vi "testmyrio.vi"() -> ()   [LabVIEW 2014]
uses:
  <vilib>/Platform/TimedLoop/XDataNode/timing_clust.ctl
  <vilib>/Platform/TimedLoop/XDataNode/nitl_modes.ctl
  <vilib>/Platform/TimedLoop/XDataNode/wakeup.ctl
  <vilib>/myRIO/Common/Instrument Driver Framework/myRIO v1.0/PWM/vis/myRIO v1.1 Open PWM.vi
  <vilib>/myRIO/Common/Instrument Driver Framework/Utilities/vis/Validate Channels.vi
  <vilib>/myRIO/Common/Instrument Driver Framework/myRIO v1.0/PWM/vis/myRIO v1.0 Reserve PWM.vi
  <vilib>/myRIO/Common/Instrument Driver Framework/myRIO v1.0/PWM/vis/myRIO v1.0 Build MUX Configuration PWM.vi
  <vilib>/myRIO/Common/Instrument Driver Framework/myRIO v1.0/Resource Manager/vis/myRIO v1.0 Reserve Channel List.vi
  <vilib>/myRIO/Common/Instrument Driver Framework/myRIO v1.0/Resource Manager/vis/myRIO v1.0 Create Configuration List.vi
  <vilib>/myRIO/Common/Instrument Driver Framework/myRIO v1.0/Resource Manager/vis/myRIO v1.0 Reserve Channel.vi
  <vilib>/myRIO/Common/Instrument Driver Framework/myRIO v1.0/Resource Manager/vis/myRIO v1.0 Unreserve Channel.vi
  <vilib>/myRIO/Common/Instrument Driver Framework/myRIO v1.0/Resource Manager/vis/myRIO v1.0 Build Mutex Name.vi
  <vilib>/Utility/VariantDataType/GetNumericInfo.vi
  <vilib>/Utility/error.llb/Error Cluster From Error Code.vi
  <vilib>/myRIO/Common/Instrument Driver Framework/myRIO v1.0/myRIO v1.1 Open.vi
  <vilib>/myRIO/Common/Instrument Driver Framework/Utilities/vis/IO Manager.vi
  <vilib>/myRIO/Common/Instrument Driver Framework/Utilities/vis/Configuration Manager.vi
  <vilib>/myRIO/Common/Instrument Driver Framework/myRIO v1.0/Resource Manager/vis/myRIO v1.0 Configure IO.vi
  <vilib>/myRIO/Common/Instrument Driver Framework/myRIO v1.0/myRIO v1.0 Close.vi
  <vilib>/Utility/AngleManip/Degrees to Radians (Scalar DBL).vi
  <vilib>/myRIO/Common/Instrument Driver Framework/myRIO v1.0/PWM/vis/myRIO v1.0 Write PWM.vi
  <vilib>/Platform/TimedLoop/XDataNode/XDataNode.xnode
  <vilib>/Platform/TimedLoop/XDataNode/XDNodeRunTimeDep.lvlib
  <vilib>/Utility/AngleManip/NI_AngleManipulation.lvlib
  <vilib>/myRIO/Instrument Drivers/Onboard IO/PWM/PWM.lvlib
panel:
  in  "Knob":dbl(knob)=125.18911398343852 scale=-180.0..180.0
  in  "open/close":dbl(slide)=-99.18367346938776 scale=-180.0..180.0
  out "theta3":dbl
  out "x/y 4":dbl
  out "x/y 3":dbl
  out "x/y 2":dbl
  out "x/y":dbl
  out "s? t:f":dbl[](array[numeric])
  in  "stop":bool
  in  "theta":dbl(knob) scale=-180.0..180.0
  in  "X":dbl(slide)=4.08910891089109 scale=0.0..11.0
  in  "Y":dbl(slide)=4.790575916230366 scale=0.0..11.9
  out "Invalid Position":bool
  out "appended array":dbl[](array[numeric])
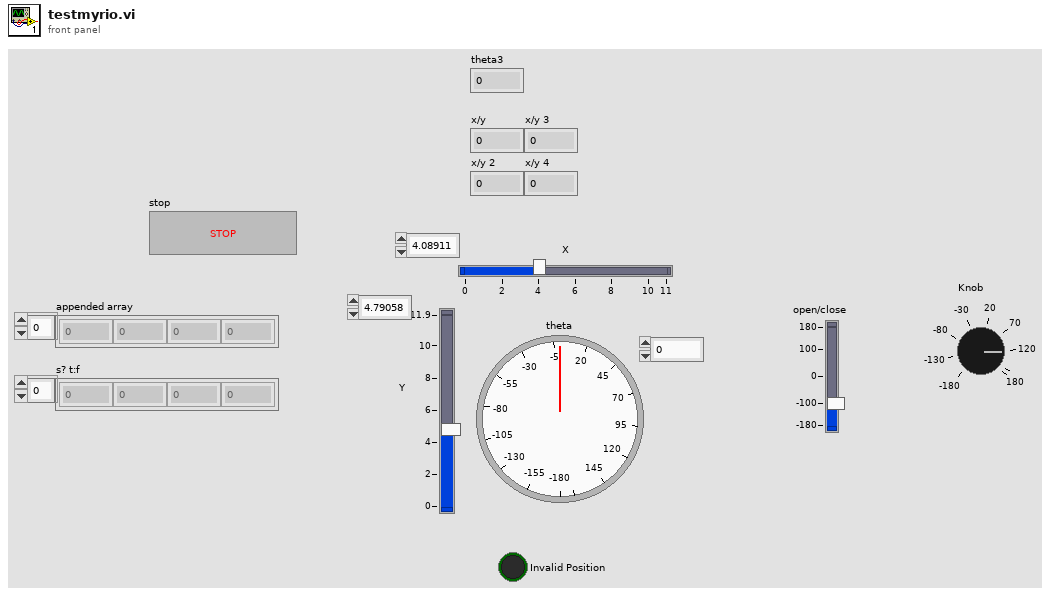
[diagram p1: front panel]
types:
  T1 = typedef "PWM.lvlib/PWM Reference.ctl" = cluster{"myRIO Reference":T2, "PWM Channels Enum":T6, "PWM Configuration":T7}
  T2 = typedef "myRIO Generic Hardware Reference.ctl" = cluster{"myRIO Model":T3, "myRIO Hardware Reference":T4}
  T3 = typedef "Hardware Version Enum.ctl" = enum16{"Unknown", "myRIO-1900", "myRIO-1950"}
  T4 = typedef "myRIO v1.0 Reference.ctl" = cluster{"Generic FPGA Reference":T5, "Allow multiple opens":bool}
  T5 = typedef "Generic FPGA Reference.ctl" = refnum<k20>
  T6 = typedef "PWM Channels Enum.ctl" = enum16{"Not Connected", "C/PWM0", "C/PWM1", "A/PWM0", "A/PWM1", "A/PWM2", "B/PWM0", "B/PWM1", "B/PWM2"}
  T7 = typedef "PWM.lvlib/PWM Configuration.ctl" = cluster{"Frequency":dbl, "Duty Cycle":dbl}
  T8 = typedef "XDNodeRunTimeDep.lvlib/timing_clust.ctl" = cluster{"Expected End [f-1]":u64, "Actual End [f-1]":u64, "Finished Late? [f-1]":bool, "Expected End [i-1]":u64, "Actual End [i-1]":u64, "Finished Late? [i-1]":bool, "Expected Start [i]":u64, "Actual Start [i]":u64, "Expected Start [f]":u64, "Actual Start [f]":u64, "Source Name":string, "Structure Name":string, "Period":i64, "Deadline":i64, "Offset":i64, "Start":i64, "Priority":i32, "Timeout":i32, "Mode":T9, "Wakeup Reason":T10, "Error":errorcluster, "Source Type":string, "Secondary Source Type":string, "Global End Time":u64, "Global Start Time":u64, "Frame Duration":u64, "Iteration Duration":u64, "Assigned CPU":i32, "I/O Scan Engine Mode":u32}
  T9 = typedef "XDNodeRunTimeDep.lvlib/nitl_modes.ctl" = enum32{"No Change", "Process missed periods, maintain original phase", "Discard missed periods, maintain original phase", "Process missed periods, ignore original phase", "Discard missed periods, ignore original phase"}
  T10 = typedef "XDNodeRunTimeDep.lvlib/wakeup.ctl" = enum32{"Normal", "Aborted", "Asynchronous wakeup", "Timing source error", "Timed loop error", "Timeout"}
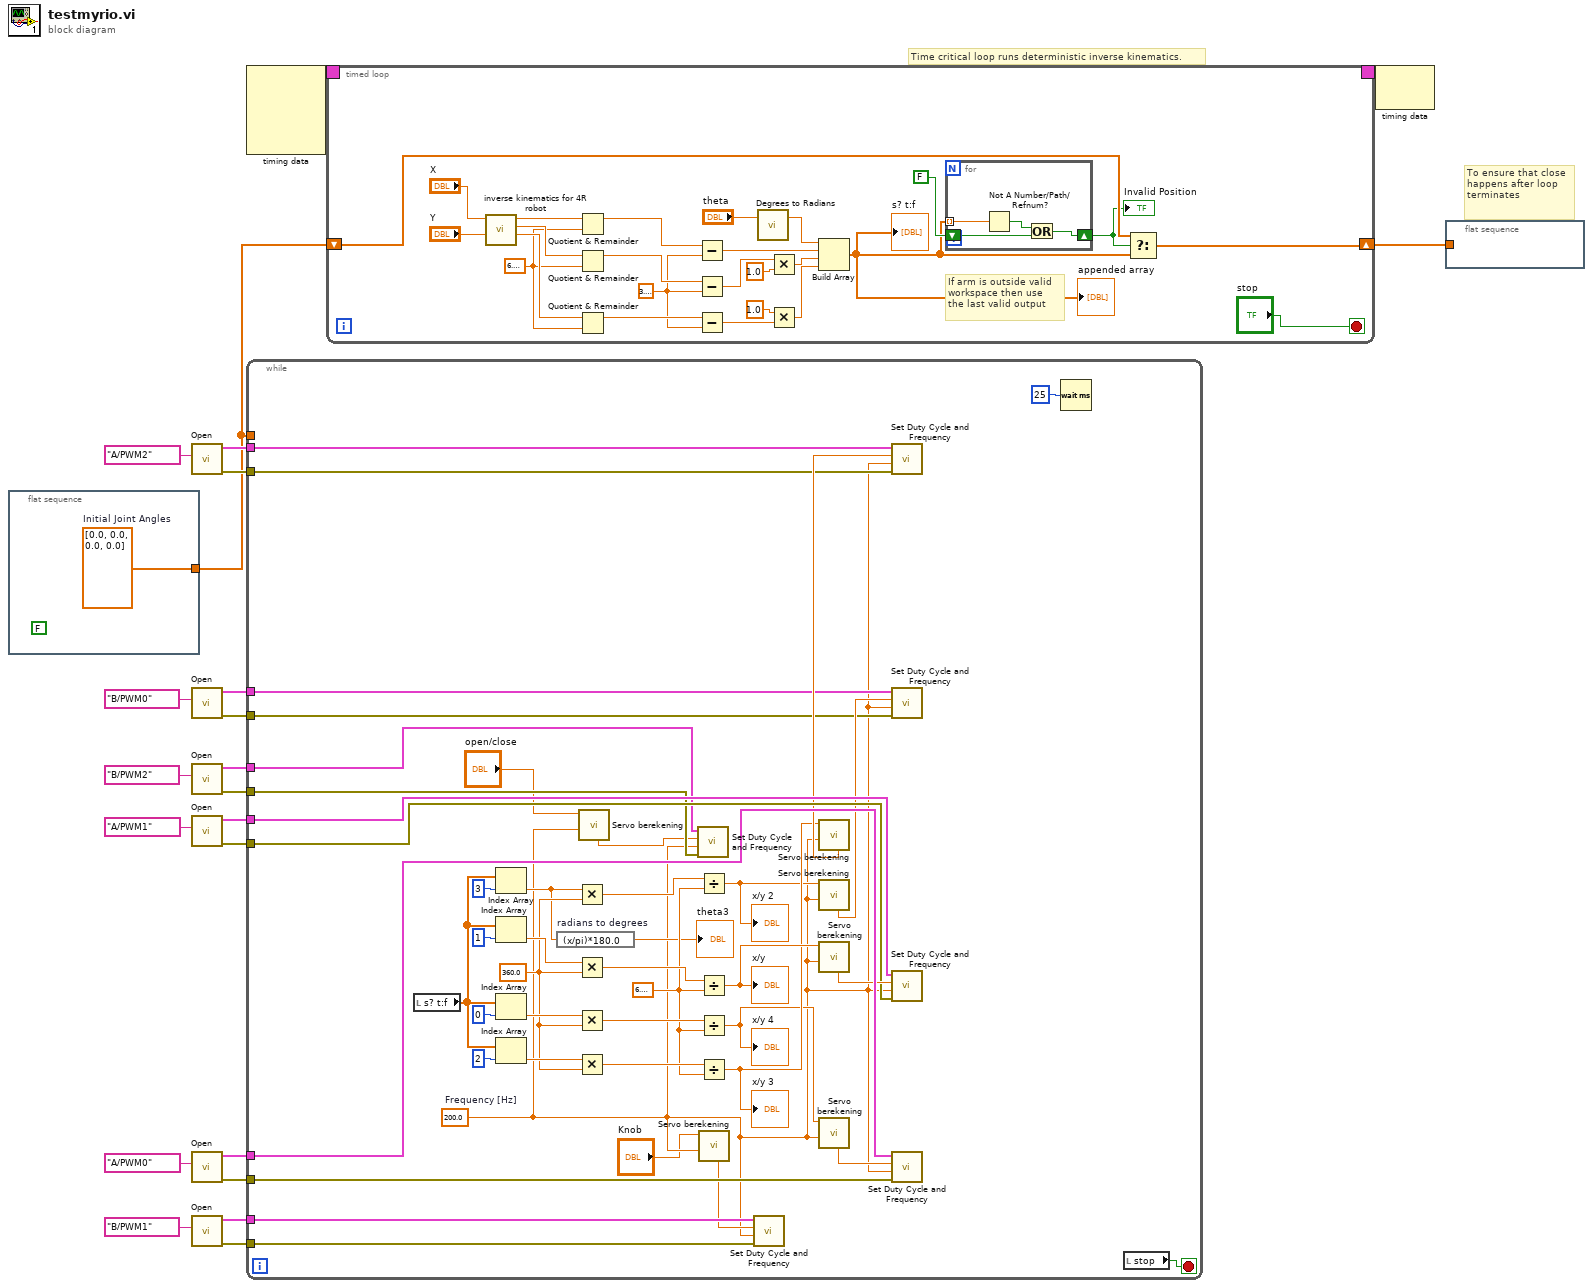
[diagram p0: block diagram]
diagram:
  # "To ensure that close happens after loop terminates"
  # "Time critical loop runs deterministic inverse kinematics."
  n1 = flat-sequence {
    tunnel: [w23] -> w7
    frame #0 {
      (unwired) FALSE ("stop")
      w23 = dbl[] [0.0, 0.0, 0.0, 0.0]  # Initial Joint Angles
    }
  }
  n2 = call <vilib>:"Open.vi"("Channel Name"=tag "A/PWM2") -> ("error out"=w11:errorcluster, "PWM Ref Out"=w12:T1)  [unwired: 9 in]
  n3 = call <vilib>:"Open.vi"("Channel Name"=tag "B/PWM0") -> ("error out"=w8:errorcluster, "PWM Ref Out"=w9:T1)  [unwired: 9 in]
  n4 = call <vilib>:"Open.vi"("Channel Name"=tag "B/PWM2") -> ("error out"=w4:errorcluster, "PWM Ref Out"=w5:T1)  [unwired: 9 in]
  n5 = call <vilib>:"Open.vi"("Channel Name"=tag "A/PWM1") -> ("error out"=w14:errorcluster, "PWM Ref Out"=w15:T1)  [unwired: 9 in]
  n6 = call <vilib>:"Open.vi"("Channel Name"=tag "A/PWM0") -> ("error out"=w18:errorcluster, "PWM Ref Out"=w19:T1)  [unwired: 9 in]
  n7 = call <vilib>:"Open.vi"("Channel Name"=tag "B/PWM1") -> ("error out"=w1:errorcluster, "PWM Ref Out"=w2:T1)  [unwired: 9 in]
  n8 = node-c288() -> (w22:T8)  [unwired: 4 in]
  n9 = while {
    tunnel: w19 -> [w62]
    tunnel: w18 -> [w61]
    tunnel: w15 -> [w59]
    tunnel: w14 -> [w58]
    tunnel: w12 -> [w55]
    tunnel: w11 -> [w54]
    tunnel: w9 -> [w51]
    tunnel: w8 -> [w50]
    tunnel: w7 -> [_]
    tunnel: w5 -> [w32]
    tunnel: w4 -> [w31]
    tunnel: w2 -> [w28]
    tunnel: w1 -> [w27]
    stop <- w33 stop-if-true
    w37 = 6.283185307179586
    w38 = 360.0 ("y")
    w25 = 200.0  # Frequency [Hz]
    n10 = local read "s? t:f"() -> (w49:dbl[])
    n11 = Index Array(array=w49, index=3) -> (element=w35:dbl)
    n12 = Index Array(array=w49, index=1) -> (element=w44:dbl)
    n13 = Index Array(array=w49, index=0) -> (element=w40:dbl)
    n14 = Index Array(array=w49, index=2) -> (element=w42:dbl)
    n15 = expression code="(x/pi)*180.0" "radians to degrees"(w35) -> (→"theta3":dbl)
    n16 = Multiply(x=w35, y=w38) -> (x*y=w46:dbl)
    n17 = Multiply(x=w44, y=w38) -> (x*y=w48:dbl)
    n18 = Multiply(x=w40, y=w38) -> (x*y=w45:dbl)
    n19 = Multiply(x=w42, y=w38) -> (x*y=w47:dbl)
    n20 = call "Servo berekening.vi"("freq [Hz]"=w25, "position [%FS] in"="open/close") -> ("Duty Cycle"=w30:dbl)  [unwired: 6 in, 3 out]
    n21 = call <vilib>:"Set Duty Cycle and Frequency.vi"("error in (no error)"=w31, "Frequency [Hz]"=w25, "Duty Cycle"=w30, "PWM Ref In"=w32) -> ()  [unwired: 5 in, 2 out]
    n22 = Divide(x=w46, y=w37) -> (x/y=w39:dbl)
    "x/y 2" <- w39
    n23 = Divide(x=w48, y=w37) -> (x/y=w43:dbl)
    "x/y" <- w43
    n24 = Divide(x=w45, y=w37) -> (x/y=w36:dbl)
    "x/y 4" <- w36
    n25 = Divide(x=w47, y=w37) -> (x/y=w41:dbl)
    "x/y 3" <- w41
    n26 = call "Servo berekening.vi"("freq [Hz]"=w25, "position [%FS] in"="Knob") -> ("Duty Cycle"=w26:dbl)  [unwired: 6 in, 3 out]
    n27 = call <vilib>:"Set Duty Cycle and Frequency.vi"("error in (no error)"=w27, "Frequency [Hz]"=w25, "Duty Cycle"=w26, "PWM Ref In"=w28) -> ()  [unwired: 5 in, 2 out]
    n28 = call "Servo berekening.vi"("freq [Hz]"=w25, "position [%FS] in"=w41) -> ("Duty Cycle"=w56:dbl)  [unwired: 6 in, 3 out]
    n29 = call "Servo berekening.vi"("freq [Hz]"=w25, "position [%FS] in"=w39) -> ("Duty Cycle"=w52:dbl)  [unwired: 6 in, 3 out]
    n30 = call "Servo berekening.vi"("freq [Hz]"=w25, "position [%FS] in"=w43) -> ("Duty Cycle"=w60:dbl)  [unwired: 6 in, 3 out]
    n31 = call "Servo berekening.vi"("freq [Hz]"=w25, "position [%FS] in"=w36) -> ("Duty Cycle"=w63:dbl)  [unwired: 6 in, 3 out]
    n32 = call <vilib>:"Set Duty Cycle and Frequency.vi"("error in (no error)"=w54, "Frequency [Hz]"=w25, "Duty Cycle"=w56, "PWM Ref In"=w55) -> ()  [unwired: 5 in, 2 out]
    n33 = call <vilib>:"Set Duty Cycle and Frequency.vi"("error in (no error)"=w50, "Frequency [Hz]"=w25, "Duty Cycle"=w52, "PWM Ref In"=w51) -> ()  [unwired: 5 in, 2 out]
    n34 = call <vilib>:"Set Duty Cycle and Frequency.vi"("error in (no error)"=w58, "Frequency [Hz]"=w25, "Duty Cycle"=w60, "PWM Ref In"=w59) -> ()  [unwired: 5 in, 2 out]
    n35 = call <vilib>:"Set Duty Cycle and Frequency.vi"("error in (no error)"=w61, "Frequency [Hz]"=w25, "Duty Cycle"=w63, "PWM Ref In"=w62) -> ()  [unwired: 5 in, 2 out]
    n36 = Wait (ms)(milliseconds to wait=u32 25) -> ()  [unwired: 1 out]
    n37 = local read "stop"() -> (w33:bool)
  }
  n38 = timed-loop {
    timing: w22 -> [_]
    timing-out: [_] -> w21
    shift-right: [w85] -> w20
    shift-left: w7 -> [w88]
    stop <- "stop" stop-if-true
    w67 = 3.141592653589793
    w75 = 6.283185307179586
    # "If arm is outside valid \nworkspace then use \nthe last valid output"
    n39 = call "inverse kinematics for 4R robot.vi"("y"="Y", "x"="X") -> ("theta3"=w77:dbl, "theta2"=w78:dbl, "theta1"=w79:dbl)  [unwired: 3 in]
    n40 = Quotient & Remainder(x=w79, y=w75) -> (x-y*floor(x/y)=w70:dbl)  [unwired: 1 out]
    n41 = Quotient & Remainder(x=w78, y=w75) -> (x-y*floor(x/y)=w72:dbl)  [unwired: 1 out]
    n42 = Quotient & Remainder(x=w77, y=w75) -> (x-y*floor(x/y)=w69:dbl)  [unwired: 1 out]
    n43 = Subtract(x=w70, y=w67) -> (x-y=w73:dbl)
    n44 = Subtract(x=w72, y=w67) -> (x-y=w71:dbl)
    n45 = Subtract(x=w69, y=w67) -> (x-y=w68:dbl)
    n46 = call-poly <vilib>:"Degrees to Radians.vi"("angle (deg)"="theta") -> ("angle (rad)"=w90:dbl)  [unwired: 2 in]
    n47 = Multiply(x=w71, y=1.0) -> (x*y=w81:dbl)
    n48 = Multiply(x=1.0, y=w68) -> (x*y=w80:dbl)
    n49 = Build Array(w90, w73, w81, w80) -> (w83:dbl[])
    "appended array" <- w83
    "s? t:f" <- w83
    n50 = for {
      tunnel: w83 -> [w95] mode=indexing
      shift-right: [w93] -> w87
      shift-left: FALSE -> [w92]
      n51 = Not A Number/Path/Refnum?(number/path/refnum=w95) -> (NaN/Path/Refnum?=w94:bool)
      n52 = Or(x=w94, y=w92) -> (x .or. y?=w93:bool)
    }
    "Invalid Position" <- w87
    n53 = Select(t=w88, s=w87, f=w83) -> (s? t:f=w85:dbl[])
  }
  n54 = node-c288(w21) -> ()  [unwired: 1 out]
  n55 = flat-sequence {
    tunnel: w20 -> [_]
    frame #0 {
    }
  }
